vi "Bundle.vi"(8 "error in (no error)":errorcluster, 10 "Driver Name":string, 11 "Reorder Driver Aliases Msg in":refnum<class "Reorder Driver Aliases Msg.lvclass">) -> (0 "error out":errorcluster, 3 "Reorder Driver Aliases Msg out":refnum<class "Reorder Driver Aliases Msg.lvclass">)   [LabVIEW 2020, in "Instrument Handler.lvlib" / "Reorder Driver Aliases Msg.lvclass"]
doc: "Populate the Reorder Driver Aliases Msg."
uses:
  Reorder Driver Aliases Msg.lvclass
  Reorder Driver Aliases Msg.lvclass/Reorder Driver Aliases Msg.ctl
panel:
  in  "New indices":u32[](array[numeric])
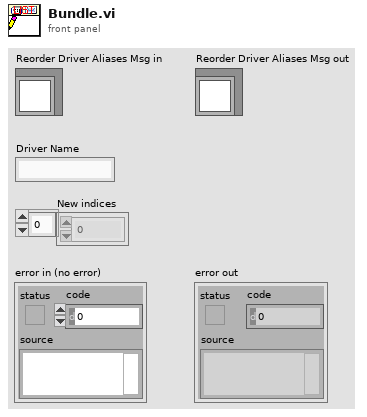
[diagram p1: front panel]
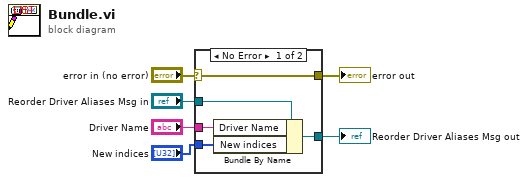
[diagram p0: block diagram]
diagram:
  n1 = case shown="No Error" "error in (no error)" {
    selector: "error in (no error)" -> [w11 w12]
    tunnel: [w11 w12] -> w5
    tunnel: [w9 w13] -> w3
    tunnel: "Reorder Driver Aliases Msg in" -> [w10 w13]
    tunnel: "Driver Name" -> [w8 _]
    tunnel: "New indices" -> [w7 _]
    frame No Error {
      n2 = Bundle By Name(cluster=w10, "Driver Name"=w8, "New indices"=w7) -> (w9:refnum<class "Reorder Driver Aliases Msg.lvclass">)
    }
    frame Error {
    }
  }
  "error out" <- w5
  "Reorder Driver Aliases Msg out" <- w3
